vi "VITester_Provider_OnUpdateCommandBegin.vi"(11 "Project Refnum":refnum<vi>) -> ()   [LabVIEW 2013]
panel:
  out "error out":errorcluster
  in  "error in":errorcluster
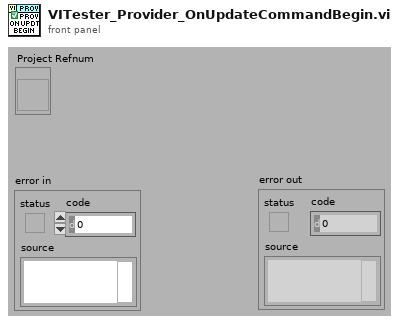
[diagram p1: front panel]
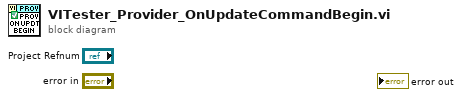
[diagram p0: block diagram]
diagram:
